vi "Extraer.vi"() -> ()   [LabVIEW 2020]
uses:
  <vilib>/httpClient/LabVIEWHTTPClient.lvlib
panel:
  out "error out":errorcluster
  out "Humedad":dbl
  out "Temperatura":dbl
  out "Fecha":string
  out "Lateral":bool
  out "Frontal":bool
  in  "stop":bool
  out "error GET":errorcluster
  out "body GET":string
  out "headers GET":string
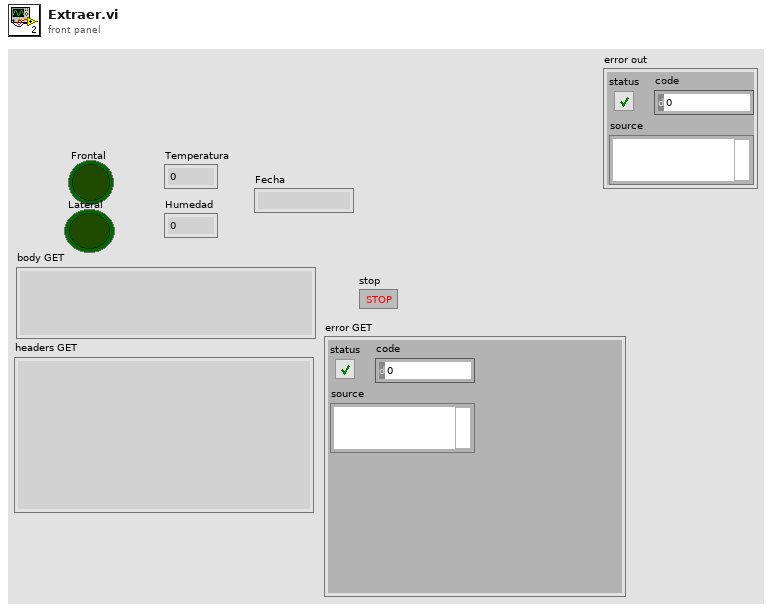
[diagram p1: front panel]
types:
  T1 = cluster{"Fecha":string, "Temperatura":dbl, "Humedad":dbl}
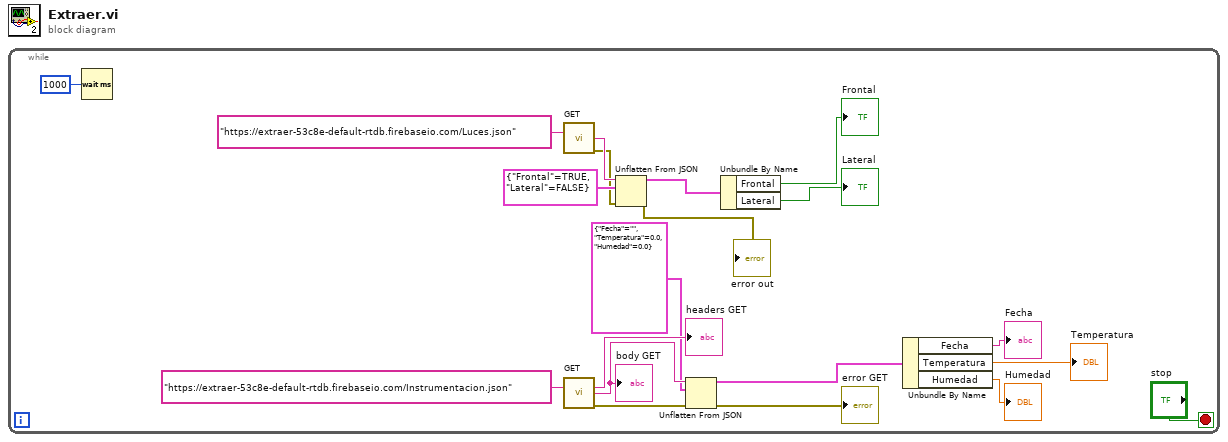
[diagram p0: block diagram]
diagram:
  n1 = while {
    stop <- "stop" stop-if-true
    n2 = Wait (ms)(milliseconds to wait=u32 1000) -> ()  [unwired: 1 out]
    n3 = call <vilib>:"GET.vi"("url"="https://extraer-53c8e-default-rtdb.firebaseio.com/Luces.json") -> ("body"=w3:string, "error out"=w2:errorcluster)  [unwired: 11 in, 2 out]
    n4 = call <vilib>:"GET.vi"("url"="https://extraer-53c8e-default-rtdb.firebaseio.com/Instrumentacion.json") -> ("headers"=→"headers GET":string, "body"=w16:string, "error out"=w15:errorcluster)  [unwired: 11 in, 1 out]
    "body GET" <- w16
    n5 = Unflatten From JSON(JSON string=w3, type and defaults=cluster{"Frontal":bool, "Lateral":bool} {"Frontal"=TRUE, "Lateral"=FALSE}, error in (no error)=w2) -> (value=w11:cluster{"Frontal":bool, "Lateral":bool}, error out=→"error out":errorcluster)  [unwired: 4 in]
    n6 = Unflatten From JSON(JSON string=w16, type and defaults=T1 {"Fecha"="", "Temperatura"=0.0, "Humedad"=0.0}, error in (no error)=w15) -> (value=w8:T1, error out=→"error GET":errorcluster)  [unwired: 4 in]
    n7 = Unbundle By Name(w11) -> ("Frontal"=→"Frontal":bool, "Lateral"=→"Lateral":bool)
    n8 = Unbundle By Name(w8) -> ("Fecha"=→"Fecha":string, "Temperatura"=→"Temperatura":dbl, "Humedad"=→"Humedad":dbl)
  }
